vi "Get Stage Values.vi"(0 "ThorlabsLTS in":refnum<class "ThorlabsLTS.lvclass">, 11 "error in (no error)":errorcluster) -> (4 "Position":dbl, 6 "Acceleration":dbl, 8 "Max velocity":dbl, 10 "Home":enum16{"off", "on"}(ring), 15 "error out 3":errorcluster)   [LabVIEW 2013, in "ThorlabsLTS.lvclass"]
uses:
  ThorlabsLTS.lvclass
  ThorlabsLTS.lvclass/ThorlabsLTS.ctl
  C:/GEECS/Developers Version/builds/Device builds/ThorLabsLTS/Thorlabs.MotionControl.IntegratedStepperMotorsCLI.dll
  Thorlabs.MotionControl.IntegratedStepperMotorsCLI.dll
  C:/GEECS/Developers Version/builds/Device builds/ThorLabsLTS/Thorlabs.MotionControl.GenericMotorCLI.dll
  Thorlabs.MotionControl.GenericMotorCLI.dll
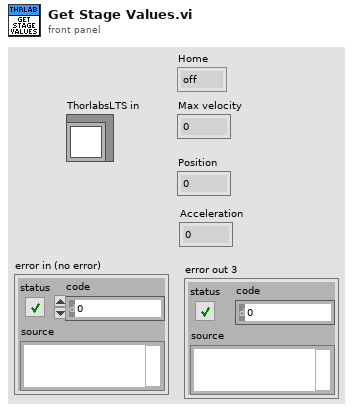
[diagram p1: front panel]
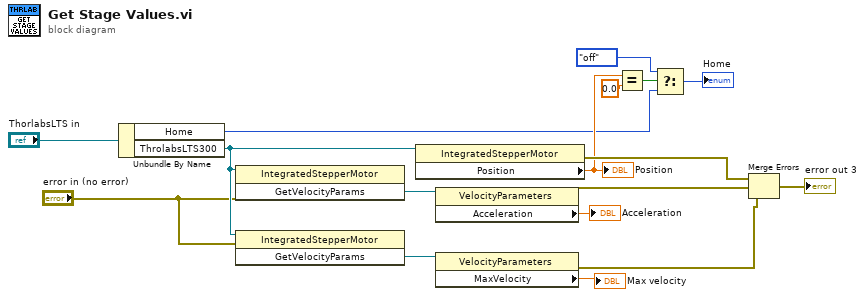
[diagram p0: block diagram]
diagram:
  n1 = Unbundle By Name ("pressure read")("ThorlabsLTS in") -> ("Home"=w3:enum16{"off", "on"}, "ThrolabsLTS300"=w17:refnum<k24>)
  n2 = invoke class="IntegratedStepperMotor" method="GetVelocityParams"(reference=w17, error in="error in (no error)") -> ("GetVelocityParams"=w15:refnum<k24>)  [unwired: 1 in, 2 out]
  n3 = invoke class="IntegratedStepperMotor" method="GetVelocityParams"(reference=w17, error in="error in (no error)") -> ("GetVelocityParams"=w16:refnum<k24>)  [unwired: 1 in, 2 out]
  n4 = property class="IntegratedStepperMotor"(reference=w17) -> (error out=w11:errorcluster, "Position"=w6:dbl)  [unwired: 1 in, 1 out]
  "Position" <- w6
  n5 = property class="VelocityParameters"(reference=w15) -> (error out=w12:errorcluster, "Acceleration"=→"Acceleration":dbl)  [unwired: 1 in, 1 out]
  n6 = property class="VelocityParameters"(reference=w16) -> (error out=w13:errorcluster, "MaxVelocity"=→"Max velocity":dbl)  [unwired: 1 in, 1 out]
  n7 = Equal?(x=w6, y=0.0) -> (x = y?=w4:bool)
  n8 = Select(t=enum16{"off", "on"}."off" ("Settings.Home"), s=w4, f=w3) -> (s? t:f=→"Home":enum16{"off", "on"})
  n9 = Merge Errors(w11, w12, w13) -> (→"error out 3":errorcluster)
